vi "Xml_Load_Sequence.vi"(7 "Version String":string, 8 "error in (no error)":errorcluster, 10 "XML Path":path=path "D:/TEST.xml", 11 "Refnum Clust":refnum<vi>) -> (0 "error out":errorcluster)   [LabVIEW 2024]
uses:
  controls/SEQUENCE_Inputs.ctl
  controls/EXCIT_Inputs.ctl
  controls/DATA_Inputs.ctl
  controls/TIMING_Inputs.ctl
  controls/PROCESSING_Inputs.ctl
  controls/TRAPPING_Inputs.ctl
  controls/RF_TRAPPING_Inputs.ctl
panel:
  in  "SEQUENCE Inputs":T1={"EXCIT Inputs"={"Number of Excitations"=1, "Script Text"="", "Table of Waveforms"=[]}, "DATA Inputs"={"Record Length"=524000, "Sample Rate"=2000000.0, "Data Type"=0, "Vertical Range"=10.0, "Acquisition Duration"=262.0}, "TIMING Inputs"={"Number of Acquisitions "=1, "Number of Accumulations"=1, "Table of Waveforms"=[], "Script Text"=""}, "PROCESSING Inputs"={"Reference Mass"=300.0939, "Cyclotron Freq"=255.727, "Magnetron Freq"=0.001}, "TRAPPING Inputs"={"Number of Channels"=4, "Init Values"=[2.0, 9.0, 2.0, 9.0], "Opening Values"=[0.0, 0.0, 0.0, 0.0], "Trapping Values"=[2.0, 9.0, 2.0, 9.0], "Emptying Values"=[-10.0, -10.0, -10.0, -10.0], "Adiabatic ON"=FALSE, "Adiabatic Duration"=100, "Adiabatic Waveforms"=["Adiabatic_None_2_2_2000", "Adiabatic_Ramp_9_0_2000", "Adiabatic_None_2_2_2000", "Adiabatic_RC_9_0_2000"], "Ions Refill ON"=FALSE, "Number of Ions Refills"=1}, "RF_TRAPPING Inputs"={"Init Values"=[0.0, 1.0, 1.0, 0.0], "Opening Values"=[0.0, -4.0, 1.0, 0.0], "Trapping Values"=[0.0, 1.0, 1.0, 0.0], "Emptying Values"=[0.0, 1.0, -7.0, 0.0], "RF Trap ON"=FALSE, "RF Accums"=1, "Number of Voltages"=4}} {"RF_TRAPPING Inputs"."RF Accums" min=1 max=100; "RF_TRAPPING Inputs"."Trapping Values" min=-10.0 max=10.0; "RF_TRAPPING Inputs"."Init Values" min=-10.0 max=10.0; "RF_TRAPPING Inputs"."Emptying Values" min=-10.0 max=10.0; "RF_TRAPPING Inputs"."Opening Values" min=-10.0 max=10.0; "TRAPPING Inputs"."Number of Ions Refills" min=1 max=1000; "TRAPPING Inputs"."Trapping Values" min=-10.0 max=10.0; "TRAPPING Inputs"."Init Values" min=-10.0 max=10.0; "TRAPPING Inputs"."Emptying Values" min=-10.0 max=10.0; "TRAPPING Inputs"."Opening Values" min=-10.0 max=10.0; "PROCESSING Inputs"."Magnetron Freq" format="%.5g"; "PROCESSING Inputs"."Cyclotron Freq" format="%.5g"; "PROCESSING Inputs"."Reference Mass" format="%.5g"; "TIMING Inputs"."Number of Accumulations" min=0 max=50 step=1; "TIMING Inputs"."Number of Acquisitions" min=1 max=10 step=1; "DATA Inputs"."Vertical Range" items=["0.2"=0.2, "0.4"=0.4, "1"=1.0, "2"=2.0, "4"=4.0, "10"=10.0]; "DATA Inputs"."Data Type" items=["I16", "DBL"]; "DATA Inputs"."Sample Rate" items=["1 MHz"=1000000.0, "2 MHz"=2000000.0, "5 MHz"=5000000.0, "10 MHz"=10000000.0, "20 MHz"=20000000.0, "25 MHz"=25000000.0, "50 MHz"=50000000.0, "100 MHz"=100000000.0]; "EXCIT Inputs"."Number of Excitations" min=1 max=10}
  # "RF_V1"
  # "RF_V2"
  # "RF_V3"
  # "RF_V4"
  # "GO_out (Trap_in_B)"
  # "Gout (Trap_out_B)"
  # "GI_in (Trap_in_A)"
  # "Gin (Trap_out_A)"
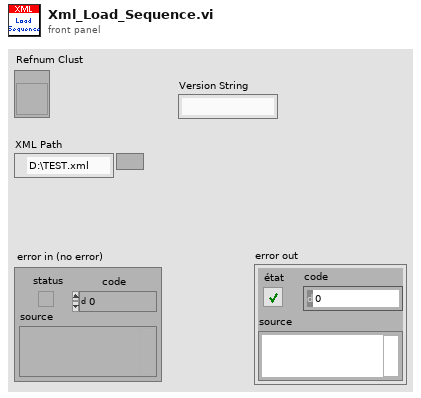
[diagram p1: front panel]
types:
  T1 = typedef "SEQUENCE_Inputs.ctl" = cluster{"EXCIT Inputs":T2, "DATA Inputs":T3, "TIMING Inputs":T4, "PROCESSING Inputs":T5, "TRAPPING Inputs":T6, "RF_TRAPPING Inputs":T7}
  T2 = typedef "EXCIT_Inputs.ctl" = cluster{"Number of Excitations":i32, "Script Text":string, "Table of Waveforms":string[]}
  T3 = typedef "DATA_Inputs.ctl" = cluster{"Record Length":i32, "Sample Rate":dbl, "Data Type":u8, "Vertical Range":dbl, "Acquisition Duration":dbl}
  T4 = typedef "TIMING_Inputs.ctl" = cluster{"Number of Acquisitions ":i16, "Number of Accumulations":i16, "Table of Waveforms":string[], "Script Text":string}
  T5 = typedef "PROCESSING_Inputs.ctl" = cluster{"Reference Mass":dbl, "Cyclotron Freq":dbl, "Magnetron Freq":dbl}
  T6 = typedef "TRAPPING_Inputs.ctl" = cluster{"Number of Channels":i32, "Init Values":dbl[], "Opening Values":dbl[], "Trapping Values":dbl[], "Emptying Values":dbl[], "Adiabatic ON":bool, "Adiabatic Duration":i32, "Adiabatic Waveforms":string[], "Ions Refill ON":bool, "Number of Ions Refills":i32}
  T7 = typedef "RF_TRAPPING_Inputs.ctl" = cluster{"Init Values":dbl[], "Opening Values":dbl[], "Trapping Values":dbl[], "Emptying Values":dbl[], "RF Trap ON":bool, "RF Accums":i32, "Number of Voltages":i32}
  T8 = cluster{"Number of Channels":i32, "Init Values":dbl[], "Opening Values":dbl[], "Trapping Values":dbl[], "Emptying Values":dbl[], "Adiabatic ON":bool, "Adiabatic Duration":i32, "Adiabatic Waveforms":string[]}
  T9 = cluster{"Number Of Acquisitions ":i16, "Number Of Accumulations":i16, "Number Of Loops":i16, "Table of Waveforms":string[], "Script text":string}
  T10 = cluster{"Record Length":i32, "Sample Rate":dbl, "Type Of Data":u8, "Vertical Range":dbl, "Acquisition Duration":dbl}
  T11 = cluster{"Number of Excitations":i32, "Script text":string, "Table of Waveforms":string[]}
  T12 = cluster{"Reference Mass":dbl, "Cyclotron Freq":dbl, "Magnetron Freq":dbl}
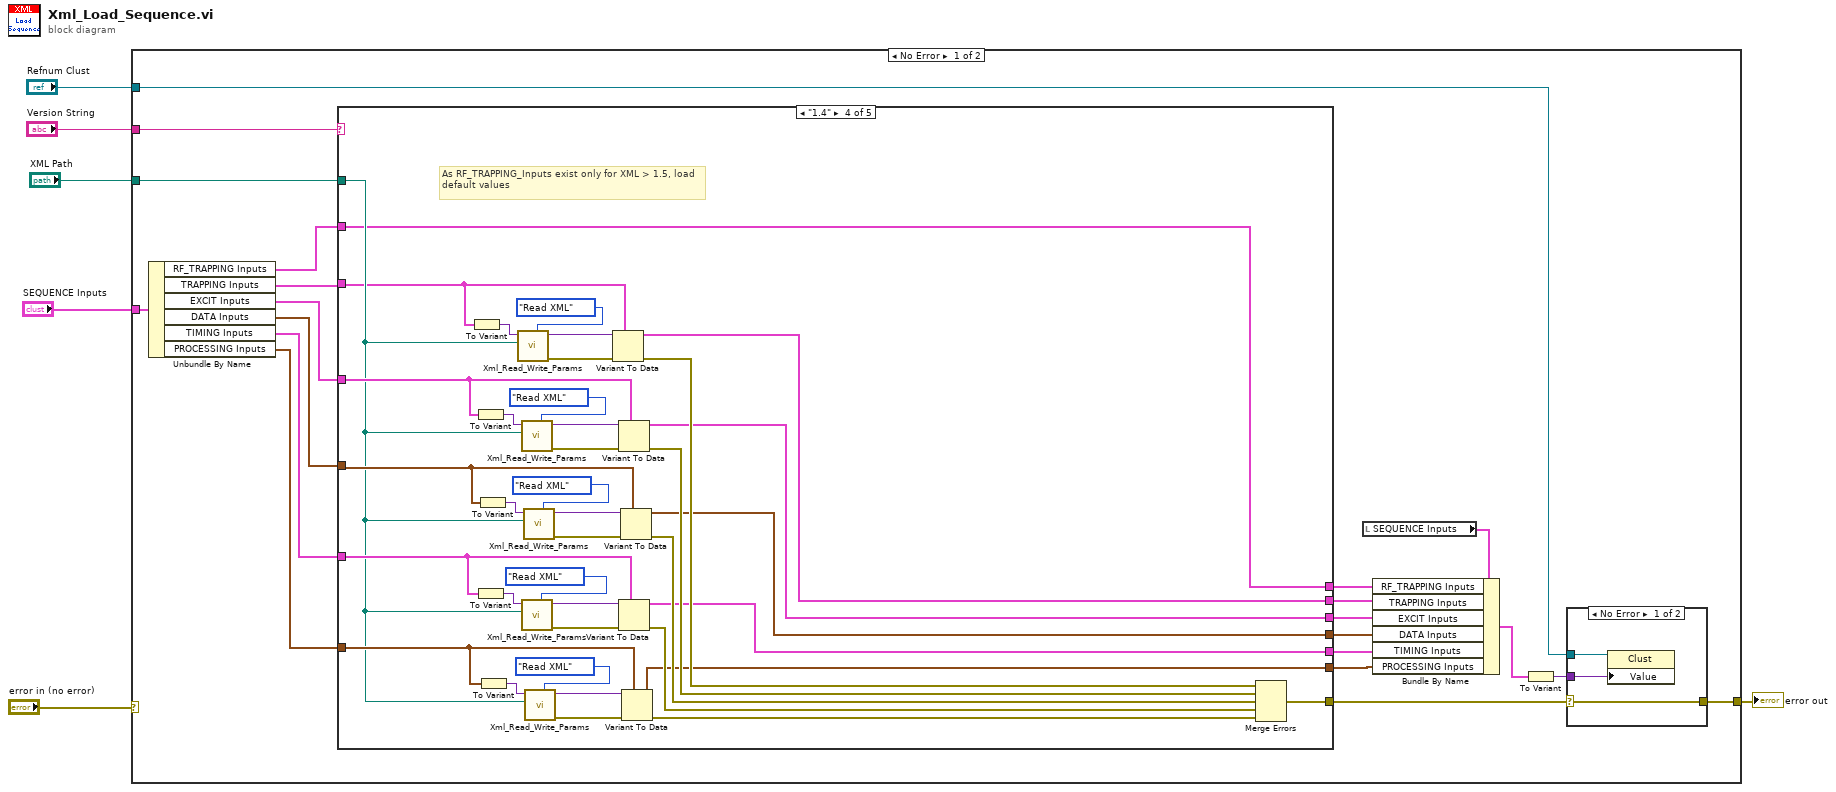
[diagram p0: block diagram]
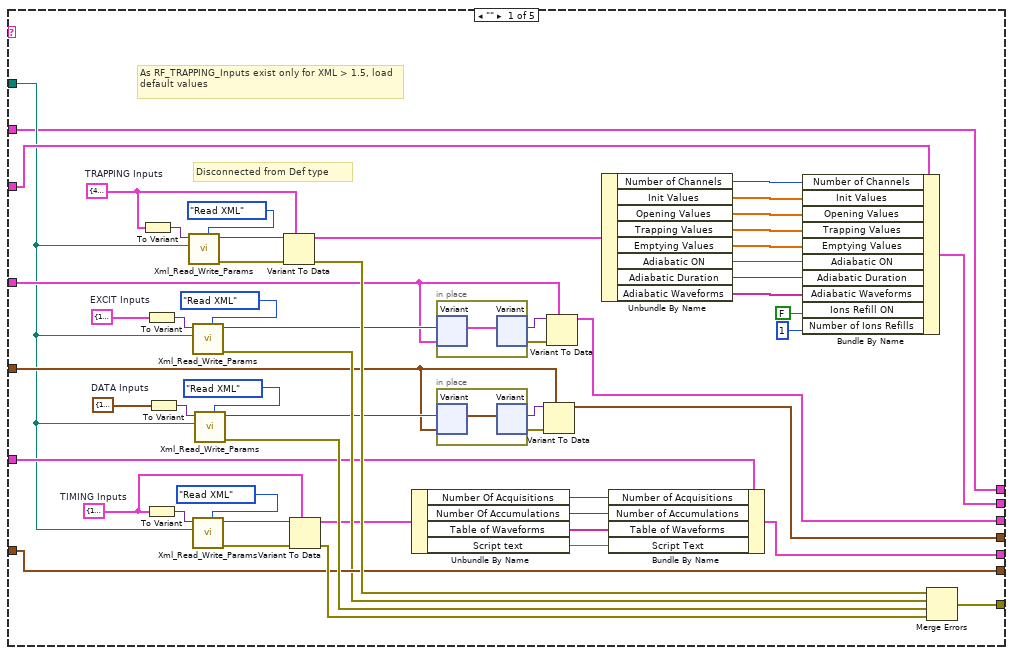
[diagram p2: hidden frame]
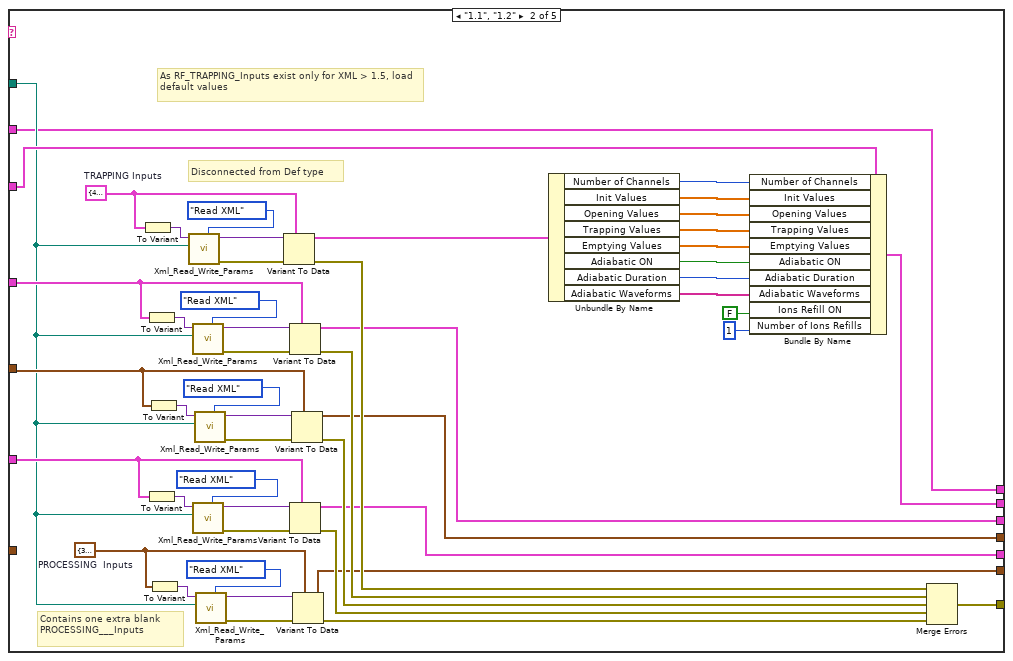
[diagram p3: hidden frame]
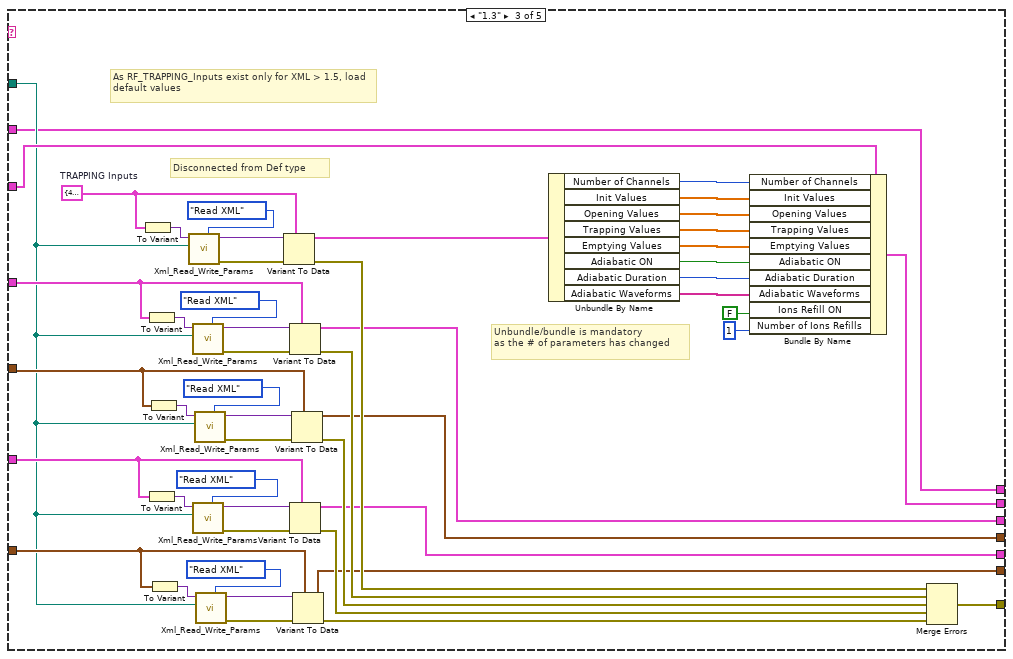
[diagram p4: hidden frame]
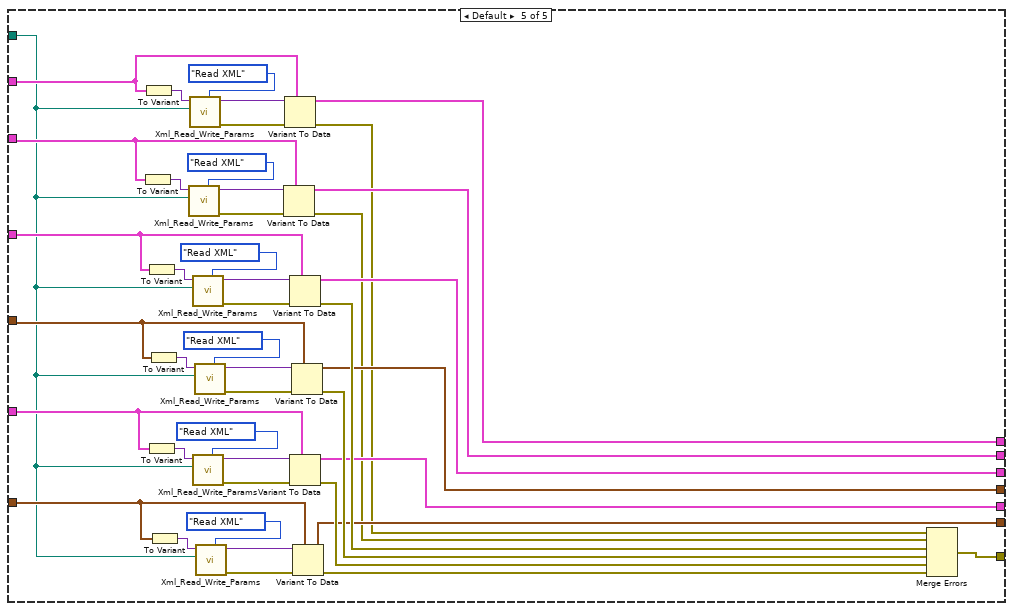
[diagram p5: hidden frame]
diagram:
  n1 = case shown="No Error" "error in (no error)" {
    selector: "error in (no error)" -> [_ w270]
    tunnel: "XML Path" -> [w27 _]
    tunnel: [w24 w270] -> w4
    tunnel: "Version String" -> [w26 _]
    tunnel: "Refnum Clust" -> [w23 _]
    tunnel: "SEQUENCE Inputs" -> [w22 _]
    frame No Error {
      n2 = Unbundle By Name(w22) -> ("RF_TRAPPING Inputs"=w8:T7, "TRAPPING Inputs"=w21:T6, "EXCIT Inputs"=w20:T2, "DATA Inputs"=w19:T3, "TIMING Inputs"=w18:T4, "PROCESSING Inputs"=w17:T5)
      n3 = case shown="\"1.4\"" w26 {
        tunnel: w27 -> [w29 w85 w135 w187 w222]
        tunnel: [w81 w133 w183 w221 w265] -> w25
        tunnel: w21 -> [w63 w97 w137 w185 w240]
        tunnel: w20 -> [w56 w107 w157 w195 w239]
        tunnel: w19 -> [w50 w106 w156 w194 w238]
        tunnel: w18 -> [w43 w105 w155 w193 w237]
        tunnel: w17 -> [w62 _ w154 w192 w236]
        tunnel: [w64 w98 w139 w184 w235] -> w16
        tunnel: [w41 w104 w153 w191 w234] -> w11
        tunnel: [w51 w103 w152 w190 w233] -> w10
        tunnel: [w42 w102 w151 w189 w232] -> w15
        tunnel: [w62 w101 w150 w188 w231] -> w14
        tunnel: w8 -> [w28 w84 w134 w186 w226]
        tunnel: [w28 w84 w134 w186 w223] -> w7
        frame "" {
          w40 = T8 {"Number of Channels"=4, "Init Values"=[2.0, 9.0, 2.0, 9.0], "Opening Values"=[0.0, 0.0, 0.0, 0.0], "Trapping Values"=[2.0, 9.0, 2.0, 9.0], "Emptying Values"=[-10.0, -10.0, -10.0, -10.0], "Adiabatic ON"=FALSE, "Adiabatic Duration"=100, "Adiabatic Waveforms"=["Adiabatic_None_2_2_2000", "Adiabatic_Ramp_9_0_2000", "Adiabatic_None_2_2_2000", "Adiabatic_RC_9_0_2000"]}  # TRAPPING Inputs
          w49 = T9 {"Number Of Acquisitions "=1, "Number Of Accumulations"=1, "Number Of Loops"=1, "Table of Waveforms"=[], "Script text"=""}  # TIMING Inputs
          w55 = T10 {"Record Length"=100000, "Sample Rate"=10000000.0, "Type Of Data"=0, "Vertical Range"=10.0, "Acquisition Duration"=100000.0}  # DATA Inputs
          w61 = T11 {"Number of Excitations"=1, "Script text"="", "Table of Waveforms"=[]}  # EXCIT Inputs
          # "As RF_TRAPPING_Inputs exist only for XML > 1.5, load default values"
          # "Disconnected from Def type"
          n4 = To Variant(anything=w40) -> (Variant=w80:variant)
          n5 = To Variant(anything=w61) -> (Variant=w75:variant)
          n6 = To Variant(anything=w49) -> (Variant=w68:variant)
          n7 = To Variant(anything=w55) -> (Variant=w74:variant)
          n8 = call "Xml_Read_Write_Params.vi"("Variant"=w80, "XML Path"=w29, "Command"=enum16{"Read XML", "Set", "Get", "Write XML"}."Read XML") -> ("Variant Output"=w78:variant, "error out"=w79:errorcluster)  [unwired: 4 in, 1 out]
          n9 = call "Xml_Read_Write_Params.vi"("Variant"=w75, "XML Path"=w29, "Command"=enum16{"Read XML", "Set", "Get", "Write XML"}."Read XML") -> ("Variant Output"=w59:variant, "error out"=w60:errorcluster)  [unwired: 4 in, 1 out]
          n10 = call "Xml_Read_Write_Params.vi"("Variant"=w68, "XML Path"=w29, "Command"=enum16{"Read XML", "Set", "Get", "Write XML"}."Read XML") -> ("Variant Output"=w70:variant, "error out"=w69:errorcluster)  [unwired: 4 in, 1 out]
          n11 = call "Xml_Read_Write_Params.vi"("Variant"=w74, "XML Path"=w29, "Command"=enum16{"Read XML", "Set", "Get", "Write XML"}."Read XML") -> ("Variant Output"=w54:variant, "error out"=w73:errorcluster)  [unwired: 4 in, 1 out]
          n12 = Variant To Data(error in=w79, type=w40, Variant=w78) -> (data=w39:T8, error out=w66:errorcluster)
          n13 = Variant To Data(error in=w69, type=w49, Variant=w70) -> (data=w44:T9, error out=w67:errorcluster)
          n14 = Unbundle By Name(w44) -> ("Number Of Acquisitions"=w48:i16, "Number Of Accumulations"=w47:i16, "Table of Waveforms"=w46:string[], "Script text"=w45:string)
          n15 = in-place "Structure Élément en place" {
            n16 = in-place-variant #1(w59, w56) -> (w83:T2)  [unwired: 1 out]
            n17 = in-place-variant #1(w83) -> (w57:variant, w58:errorcluster)
          }
          n18 = in-place "Structure Élément en place" {
            n19 = in-place-variant #2(w54, w50) -> (w82:T3)  [unwired: 1 out]
            n20 = in-place-variant #2(w82) -> (w52:variant, w53:errorcluster)
          }
          n21 = Variant To Data(error in=w53, type=w50, Variant=w52) -> (data=w51:T3)  [unwired: 1 out]
          n22 = Variant To Data(error in=w58, type=w56, Variant=w57) -> (data=w41:T2)  [unwired: 1 out]
          n23 = Unbundle By Name(w39) -> ("Number of Channels"=w38:i32, "Init Values"=w37:dbl[], "Opening Values"=w36:dbl[], "Trapping Values"=w35:dbl[], "Emptying Values"=w34:dbl[], "Adiabatic ON"=w31:bool, "Adiabatic Duration"=w30:i32, "Adiabatic Waveforms"=w33:string[])
          n24 = Bundle By Name(cluster=w43, "Number of Acquisitions"=w48, "Number of Accumulations"=w47, "Table of Waveforms"=w46, "Script Text"=w45) -> (w42:T4)
          n25 = Bundle By Name(cluster=w63, "Number of Channels"=w38, "Init Values"=w37, "Opening Values"=w36, "Trapping Values"=w35, "Emptying Values"=w34, "Adiabatic ON"=w31, "Adiabatic Duration"=w30, "Adiabatic Waveforms"=w33, "Ions Refill ON"=FALSE ("Ions Accumulation ON"), "Number of Ions Refills"=1) -> (w64:T6)
          n26 = Merge Errors(w66, w60, w73, w67) -> (w81:errorcluster)
        }
        frame "1.1", "1.2" {
          w95 = T8 {"Number of Channels"=4, "Init Values"=[2.0, 9.0, 2.0, 9.0], "Opening Values"=[0.0, 0.0, 0.0, 0.0], "Trapping Values"=[2.0, 9.0, 2.0, 9.0], "Emptying Values"=[-10.0, -10.0, -10.0, -10.0], "Adiabatic ON"=FALSE, "Adiabatic Duration"=100, "Adiabatic Waveforms"=["Adiabatic_None_2_2_2000", "Adiabatic_Ramp_9_0_2000", "Adiabatic_None_2_2_2000", "Adiabatic_RC_9_0_2000"]}  # TRAPPING Inputs
          w96 = T12 {"Reference Mass"=300.0939, "Cyclotron Freq"=255.727, "Magnetron Freq"=0.001}  # PROCESSING  Inputs
          # "As RF_TRAPPING_Inputs exist only for XML > 1.5, load default values"
          # "Contains one extra blank\nPROCESSING___Inputs"
          # "Disconnected from Def type"
          n27 = To Variant(anything=w95) -> (Variant=w132:variant)
          n28 = To Variant(anything=w107) -> (Variant=w125:variant)
          n29 = To Variant(anything=w105) -> (Variant=w117:variant)
          n30 = To Variant(anything=w106) -> (Variant=w124:variant)
          n31 = To Variant(anything=w96) -> (Variant=w112:variant)
          n32 = call "Xml_Read_Write_Params.vi"("Variant"=w132, "XML Path"=w85, "Command"=enum16{"Read XML", "Set", "Get", "Write XML"}."Read XML") -> ("Variant Output"=w130:variant, "error out"=w131:errorcluster)  [unwired: 4 in, 1 out]
          n33 = call "Xml_Read_Write_Params.vi"("Variant"=w125, "XML Path"=w85, "Command"=enum16{"Read XML", "Set", "Get", "Write XML"}."Read XML") -> ("Variant Output"=w127:variant, "error out"=w126:errorcluster)  [unwired: 4 in, 1 out]
          n34 = call "Xml_Read_Write_Params.vi"("Variant"=w117, "XML Path"=w85, "Command"=enum16{"Read XML", "Set", "Get", "Write XML"}."Read XML") -> ("Variant Output"=w119:variant, "error out"=w118:errorcluster)  [unwired: 4 in, 1 out]
          n35 = call "Xml_Read_Write_Params.vi"("Variant"=w124, "XML Path"=w85, "Command"=enum16{"Read XML", "Set", "Get", "Write XML"}."Read XML") -> ("Variant Output"=w122:variant, "error out"=w123:errorcluster)  [unwired: 4 in, 1 out]
          n36 = call "Xml_Read_Write_Params.vi"("Variant"=w112, "XML Path"=w85, "Command"=enum16{"Read XML", "Set", "Get", "Write XML"}."Read XML") -> ("Variant Output"=w110:variant, "error out"=w111:errorcluster)  [unwired: 4 in, 1 out]
          n37 = Variant To Data(error in=w131, type=w95, Variant=w130) -> (data=w94:T8, error out=w113:errorcluster)
          n38 = Variant To Data(error in=w126, type=w107, Variant=w127) -> (data=w104:T2, error out=w114:errorcluster)
          n39 = Variant To Data(error in=w118, type=w105, Variant=w119) -> (data=w102:T4, error out=w116:errorcluster)
          n40 = Variant To Data(error in=w123, type=w106, Variant=w122) -> (data=w103:T3, error out=w115:errorcluster)
          n41 = Variant To Data(error in=w111, type=w96, Variant=w110) -> (data=w101:T12, error out=w108:errorcluster)
          n42 = Unbundle By Name(w94) -> ("Number of Channels"=w93:i32, "Init Values"=w92:dbl[], "Opening Values"=w91:dbl[], "Trapping Values"=w90:dbl[], "Emptying Values"=w89:dbl[], "Adiabatic ON"=w88:bool, "Adiabatic Duration"=w87:i32, "Adiabatic Waveforms"=w86:string[])
          n43 = Bundle By Name(cluster=w97, "Number of Channels"=w93, "Init Values"=w92, "Opening Values"=w91, "Trapping Values"=w90, "Emptying Values"=w89, "Adiabatic ON"=w88, "Adiabatic Duration"=w87, "Adiabatic Waveforms"=w86, "Ions Refill ON"=FALSE ("Ions Accumulation ON"), "Number of Ions Refills"=1) -> (w98:T6)
          n44 = Merge Errors(w113, w114, w115, w116, w108) -> (w133:errorcluster)
        }
        frame "1.3" {
          w138 = T8 {"Number of Channels"=4, "Init Values"=[2.0, 9.0, 2.0, 9.0], "Opening Values"=[0.0, 0.0, 0.0, 0.0], "Trapping Values"=[2.0, 9.0, 2.0, 9.0], "Emptying Values"=[-10.0, -10.0, -10.0, -10.0], "Adiabatic ON"=FALSE, "Adiabatic Duration"=100, "Adiabatic Waveforms"=["Adiabatic_None_2_2_2000", "Adiabatic_Ramp_9_0_2000", "Adiabatic_None_2_2_2000", "Adiabatic_RC_9_0_2000"]}  # TRAPPING Inputs
          # "As RF_TRAPPING_Inputs exist only for XML > 1.5, load default values"
          # "Disconnected from Def type"
          # "Unbundle/bundle is mandatory\nas the # of parameters has changed"
          n45 = To Variant(anything=w138) -> (Variant=w182:variant)
          n46 = To Variant(anything=w157) -> (Variant=w175:variant)
          n47 = To Variant(anything=w155) -> (Variant=w167:variant)
          n48 = To Variant(anything=w156) -> (Variant=w174:variant)
          n49 = To Variant(anything=w154) -> (Variant=w162:variant)
          n50 = call "Xml_Read_Write_Params.vi"("Variant"=w182, "XML Path"=w135, "Command"=enum16{"Read XML", "Set", "Get", "Write XML"}."Read XML") -> ("Variant Output"=w180:variant, "error out"=w181:errorcluster)  [unwired: 4 in, 1 out]
          n51 = call "Xml_Read_Write_Params.vi"("Variant"=w175, "XML Path"=w135, "Command"=enum16{"Read XML", "Set", "Get", "Write XML"}."Read XML") -> ("Variant Output"=w177:variant, "error out"=w176:errorcluster)  [unwired: 4 in, 1 out]
          n52 = call "Xml_Read_Write_Params.vi"("Variant"=w167, "XML Path"=w135, "Command"=enum16{"Read XML", "Set", "Get", "Write XML"}."Read XML") -> ("Variant Output"=w169:variant, "error out"=w168:errorcluster)  [unwired: 4 in, 1 out]
          n53 = call "Xml_Read_Write_Params.vi"("Variant"=w174, "XML Path"=w135, "Command"=enum16{"Read XML", "Set", "Get", "Write XML"}."Read XML") -> ("Variant Output"=w172:variant, "error out"=w173:errorcluster)  [unwired: 4 in, 1 out]
          n54 = call "Xml_Read_Write_Params.vi"("Variant"=w162, "XML Path"=w135, "Command"=enum16{"Read XML", "Set", "Get", "Write XML"}."Read XML") -> ("Variant Output"=w160:variant, "error out"=w161:errorcluster)  [unwired: 4 in, 1 out]
          n55 = Variant To Data(error in=w181, type=w138, Variant=w180) -> (data=w140:T8, error out=w163:errorcluster)
          n56 = Variant To Data(error in=w176, type=w157, Variant=w177) -> (data=w153:T2, error out=w164:errorcluster)
          n57 = Variant To Data(error in=w168, type=w155, Variant=w169) -> (data=w151:T4, error out=w166:errorcluster)
          n58 = Variant To Data(error in=w173, type=w156, Variant=w172) -> (data=w152:T3, error out=w165:errorcluster)
          n59 = Variant To Data(error in=w161, type=w154, Variant=w160) -> (data=w150:T5, error out=w158:errorcluster)
          n60 = Unbundle By Name(w140) -> ("Number of Channels"=w149:i32, "Init Values"=w148:dbl[], "Opening Values"=w147:dbl[], "Trapping Values"=w146:dbl[], "Emptying Values"=w145:dbl[], "Adiabatic ON"=w144:bool, "Adiabatic Duration"=w143:i32, "Adiabatic Waveforms"=w142:string[])
          n61 = Bundle By Name(cluster=w137, "Number of Channels"=w149, "Init Values"=w148, "Opening Values"=w147, "Trapping Values"=w146, "Emptying Values"=w145, "Adiabatic ON"=w144, "Adiabatic Duration"=w143, "Adiabatic Waveforms"=w142, "Ions Refill ON"=FALSE ("Ions Accumulation ON"), "Number of Ions Refills"=1) -> (w139:T6)
          n62 = Merge Errors(w163, w164, w165, w166, w158) -> (w183:errorcluster)
        }
        frame "1.4" {
          # "As RF_TRAPPING_Inputs exist only for XML > 1.5, load default values"
          n63 = To Variant(anything=w185) -> (Variant=w220:variant)
          n64 = To Variant(anything=w195) -> (Variant=w213:variant)
          n65 = To Variant(anything=w193) -> (Variant=w205:variant)
          n66 = To Variant(anything=w194) -> (Variant=w212:variant)
          n67 = To Variant(anything=w192) -> (Variant=w200:variant)
          n68 = call "Xml_Read_Write_Params.vi"("Variant"=w220, "XML Path"=w187, "Command"=enum16{"Read XML", "Set", "Get", "Write XML"}."Read XML") -> ("Variant Output"=w218:variant, "error out"=w219:errorcluster)  [unwired: 4 in, 1 out]
          n69 = call "Xml_Read_Write_Params.vi"("Variant"=w213, "XML Path"=w187, "Command"=enum16{"Read XML", "Set", "Get", "Write XML"}."Read XML") -> ("Variant Output"=w215:variant, "error out"=w214:errorcluster)  [unwired: 4 in, 1 out]
          n70 = call "Xml_Read_Write_Params.vi"("Variant"=w205, "XML Path"=w187, "Command"=enum16{"Read XML", "Set", "Get", "Write XML"}."Read XML") -> ("Variant Output"=w207:variant, "error out"=w206:errorcluster)  [unwired: 4 in, 1 out]
          n71 = call "Xml_Read_Write_Params.vi"("Variant"=w212, "XML Path"=w187, "Command"=enum16{"Read XML", "Set", "Get", "Write XML"}."Read XML") -> ("Variant Output"=w210:variant, "error out"=w211:errorcluster)  [unwired: 4 in, 1 out]
          n72 = call "Xml_Read_Write_Params.vi"("Variant"=w200, "XML Path"=w187, "Command"=enum16{"Read XML", "Set", "Get", "Write XML"}."Read XML") -> ("Variant Output"=w198:variant, "error out"=w199:errorcluster)  [unwired: 4 in, 1 out]
          n73 = Variant To Data(error in=w219, type=w185, Variant=w218) -> (data=w184:T6, error out=w201:errorcluster)
          n74 = Variant To Data(error in=w214, type=w195, Variant=w215) -> (data=w191:T2, error out=w202:errorcluster)
          n75 = Variant To Data(error in=w206, type=w193, Variant=w207) -> (data=w189:T4, error out=w204:errorcluster)
          n76 = Variant To Data(error in=w211, type=w194, Variant=w210) -> (data=w190:T3, error out=w203:errorcluster)
          n77 = Variant To Data(error in=w199, type=w192, Variant=w198) -> (data=w188:T5, error out=w196:errorcluster)
          n78 = Merge Errors(w201, w202, w203, w204, w196) -> (w221:errorcluster)
        }
        frame Default {
          n79 = To Variant(anything=w240) -> (Variant=w264:variant)
          n80 = To Variant(anything=w226) -> (Variant=w230:variant)
          n81 = To Variant(anything=w239) -> (Variant=w257:variant)
          n82 = To Variant(anything=w237) -> (Variant=w249:variant)
          n83 = To Variant(anything=w238) -> (Variant=w256:variant)
          n84 = To Variant(anything=w236) -> (Variant=w245:variant)
          n85 = call "Xml_Read_Write_Params.vi"("Variant"=w264, "XML Path"=w222, "Command"=enum16{"Read XML", "Set", "Get", "Write XML"}."Read XML") -> ("Variant Output"=w262:variant, "error out"=w263:errorcluster)  [unwired: 4 in, 1 out]
          n86 = call "Xml_Read_Write_Params.vi"("Variant"=w230, "XML Path"=w222, "Command"=enum16{"Read XML", "Set", "Get", "Write XML"}."Read XML") -> ("Variant Output"=w228:variant, "error out"=w229:errorcluster)  [unwired: 4 in, 1 out]
          n87 = call "Xml_Read_Write_Params.vi"("Variant"=w257, "XML Path"=w222, "Command"=enum16{"Read XML", "Set", "Get", "Write XML"}."Read XML") -> ("Variant Output"=w259:variant, "error out"=w258:errorcluster)  [unwired: 4 in, 1 out]
          n88 = call "Xml_Read_Write_Params.vi"("Variant"=w249, "XML Path"=w222, "Command"=enum16{"Read XML", "Set", "Get", "Write XML"}."Read XML") -> ("Variant Output"=w251:variant, "error out"=w250:errorcluster)  [unwired: 4 in, 1 out]
          n89 = call "Xml_Read_Write_Params.vi"("Variant"=w256, "XML Path"=w222, "Command"=enum16{"Read XML", "Set", "Get", "Write XML"}."Read XML") -> ("Variant Output"=w254:variant, "error out"=w255:errorcluster)  [unwired: 4 in, 1 out]
          n90 = call "Xml_Read_Write_Params.vi"("Variant"=w245, "XML Path"=w222, "Command"=enum16{"Read XML", "Set", "Get", "Write XML"}."Read XML") -> ("Variant Output"=w243:variant, "error out"=w244:errorcluster)  [unwired: 4 in, 1 out]
          n91 = Variant To Data(error in=w263, type=w240, Variant=w262) -> (data=w235:T6, error out=w225:errorcluster)
          n92 = Variant To Data(error in=w229, type=w226, Variant=w228) -> (data=w223:T7, error out=w224:errorcluster)
          n93 = Variant To Data(error in=w258, type=w239, Variant=w259) -> (data=w234:T2, error out=w246:errorcluster)
          n94 = Variant To Data(error in=w250, type=w237, Variant=w251) -> (data=w232:T4, error out=w248:errorcluster)
          n95 = Variant To Data(error in=w255, type=w238, Variant=w254) -> (data=w233:T3, error out=w247:errorcluster)
          n96 = Variant To Data(error in=w244, type=w236, Variant=w243) -> (data=w231:T5, error out=w241:errorcluster)
          n97 = Merge Errors(w224, w225, w246, w247, w248, w241) -> (w265:errorcluster)
        }
      }
      n98 = local read "SEQUENCE Inputs"() -> (w9:T1)
      n99 = Bundle By Name(cluster=w9, "RF_TRAPPING Inputs"=w7, "TRAPPING Inputs"=w16, "EXCIT Inputs"=w11, "DATA Inputs"=w10, "TIMING Inputs"=w15, "PROCESSING Inputs"=w14) -> (w13:T1)
      n100 = To Variant(anything=w13) -> (Variant=w12:variant)
      n101 = case shown="No Error" w25 {
        selector: w25 -> [w267 w269]
        tunnel: w23 -> [w268 _]
        tunnel: [w267 w269] -> w24
        tunnel: w12 -> [w266 _]
        frame No Error {
          n102 = property class="Clust"(reference=w268, "Value"=w266) -> ()  [unwired: 1 in, 2 out]
        }
        frame Error {
        }
      }
    }
    frame Error {
    }
  }
  "error out" <- w4
